vi "Untitled 2.vi"() -> ()   [LabVIEW 2015]
panel:
  in  "Numeric":i32
  out "Array":void[](array[numeric])
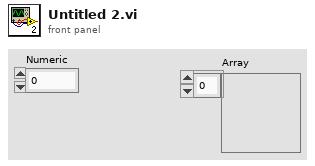
[diagram p1: front panel]
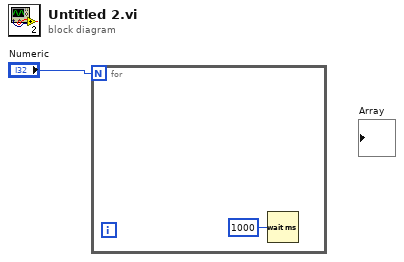
[diagram p0: block diagram]
diagram:
  n1 = for {
    N: "Numeric" -> [_]
    n2 = Wait (ms)(milliseconds to wait=u32 1000) -> ()  [unwired: 1 out]
  }
